vi "getCommentFromXml.vi"(8 "error in (no error)":errorcluster, 10 "Xml":refnum<class "xmlNode.lvclass">, 11 "ScriptEvent in":refnum<class "ScriptEvent.lvclass">) -> (0 "error out":errorcluster, 2 "Xml out":refnum<class "xmlNode.lvclass">, 3 "ScriptEvent out":refnum<class "ScriptEvent.lvclass">)   [LabVIEW 2009, in "Tools.lvlib" / "Scripting.lvlib" / "ScriptEvent.lvclass"]
uses:
  ScriptEvent.lvclass
  xmlNode/xmlNode.lvclass
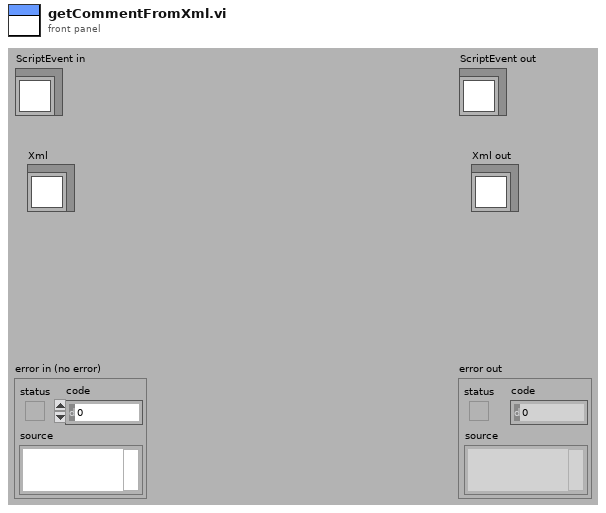
[diagram p1: front panel]
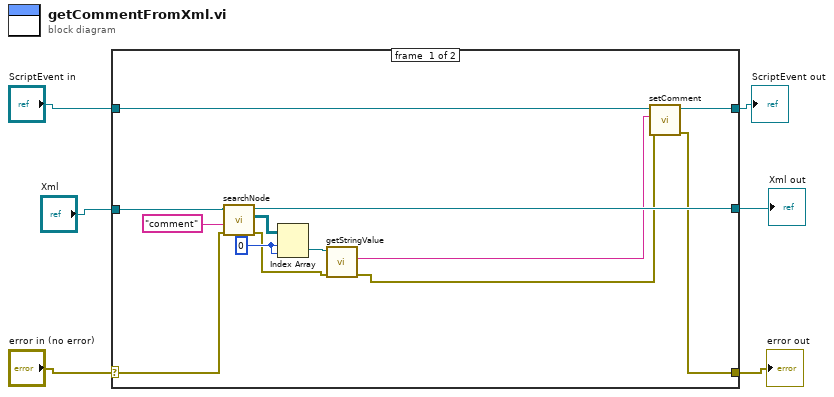
[diagram p0: block diagram]
diagram:
  n1 = case shown="No Error" "error in (no error)" {
    selector: "error in (no error)" -> [w13 w21]
    tunnel: [w7 w21] -> w1
    tunnel: [w9 w20] -> w2
    tunnel: "ScriptEvent in" -> [w11 w20]
    tunnel: "Xml" -> [w15 _]
    tunnel: [w14 _] -> w3
    frame #0 {
      w17 = 0
      n2 = call-dynamic "searchNode.vi"("error in (no error)"=w13, "searchElementName"="comment", "xmlNode in"=w15) -> ("error out"=w12:errorcluster, "arrayXmlNodes"=w18:refnum<class "xmlNode.lvclass">[][], "xmlNode out"=w14:refnum<class "xmlNode.lvclass">)  [unwired: 6 in]
      n3 = Index Array(array=w18, index (row)=w17, index (col)=w17) -> (element=w16:refnum<class "xmlNode.lvclass">)
      n4 = call-dynamic "getStringValue.vi"("error in (no error)"=w12, "xmlNode.lvclass in"=w16) -> ("error out"=w8:errorcluster, "stringValue"=w10:string)  [unwired: 7 in, 1 out]
      n5 = call-dynamic "setComment.vi"("error in (no error)"=w8, "comment"=w10, "ScriptEvent.lvclass in"=w11) -> ("error out"=w7:errorcluster, "ScriptEvent.lvclass out"=w9:refnum<class "ScriptEvent.lvclass">)  [unwired: 7 in]
    }
    frame #1 {
    }
  }
  "error out" <- w1
  "ScriptEvent out" <- w2
  "Xml out" <- w3
